vi "parse alarms string.vi"(0 "Alarms String":string) -> (4 "Description":string[](array[string]), 5 "Date":string[](array[string]), 6 "Alarm Level":string[](array[string]), 7 "Alarmed Variables":string[](array[string]), 8 "Alarmed Variable Value":string[](array[string]))   [LabVIEW 2013]
panel:
  out "Array":string[](array[string])
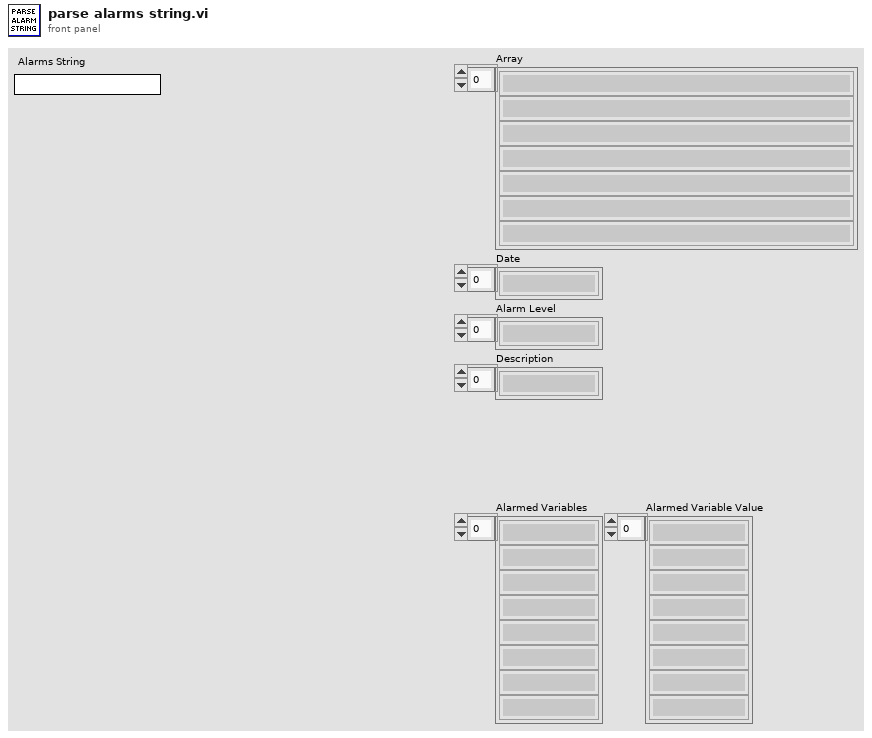
[diagram p1: front panel]
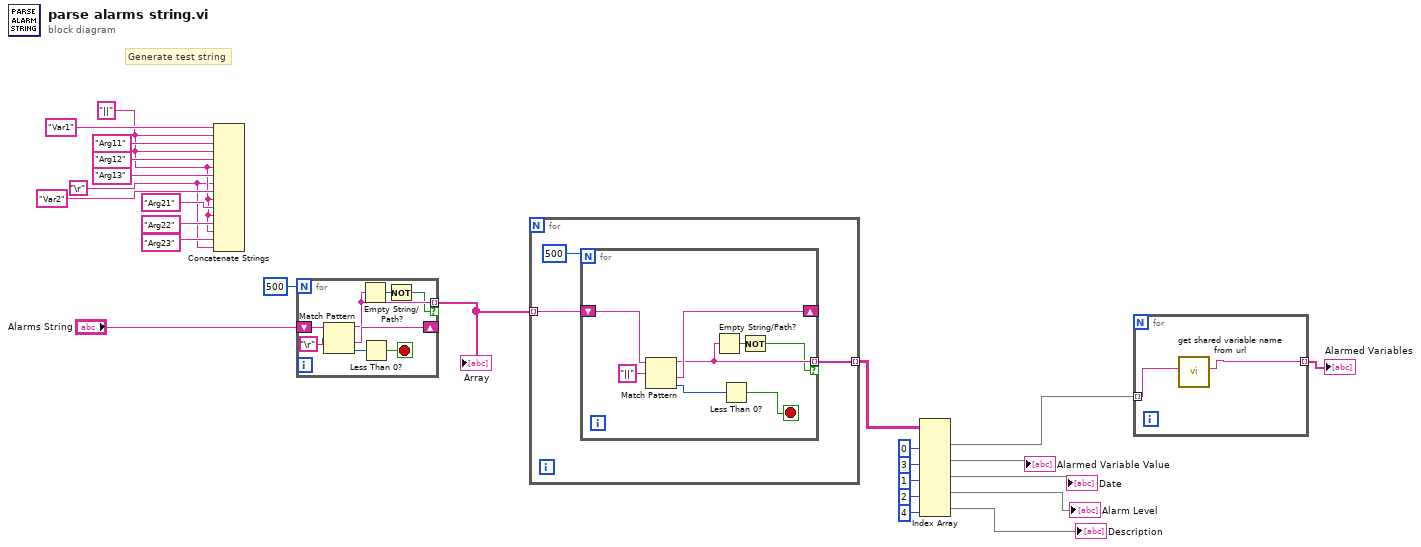
[diagram p0: block diagram]
diagram:
  w17 = "||"
  w15 = "\r"
  # "Generate test string"
  n1 = Concatenate Strings("Var1" ("string"), w17, "Arg11" ("string"), w17, "Arg12" ("string"), w17, "Arg13" ("string"), w15, "Var2" ("string"), w17, "Arg21" ("string"), w17, "Arg22" ("string"), w17, "Arg23" ("string"), w15) -> ()  [unwired: 1 out]
  n2 = for {
    N: 500 -> [_]
    shift-right: [w30] -> _
    shift-left: "Alarms String" -> [w33]
    tunnel: [w27] -> w25 mode=indexing if=w26
    stop <- w31 stop-if-true
    n3 = Match Pattern(string=w33, regular expression="\r") -> (before substring=w27:string, after substring=w30:string, offset past match=w32:i32)  [unwired: 1 in, 1 out]
    n4 = Empty String/Path?(string/path=w27) -> (empty?=w28:bool)
    n5 = Less Than 0?(x=w32) -> (x < 0?=w31:bool)
    n6 = Not(x=w28) -> (.not. x?=w26:bool)
  }
  "Array" <- w25
  n7 = for {
    tunnel: w25 -> [w36] mode=indexing
    tunnel: [w34] -> w13 mode=indexing
    n8 = for {
      N: 500 -> [_]
      shift-right: [w40] -> _
      shift-left: w36 -> [w44]
      tunnel: [w39] -> w34 mode=indexing if=w37
      stop <- w41 stop-if-true
      n9 = Match Pattern(string=w44, regular expression="||") -> (before substring=w39:string, after substring=w40:string, offset past match=w42:i32)  [unwired: 1 in, 1 out]
      n10 = Empty String/Path?(string/path=w39) -> (empty?=w38:bool)
      n11 = Less Than 0?(x=w42) -> (x < 0?=w41:bool)
      n12 = Not(x=w38) -> (.not. x?=w37:bool)
    }
  }
  n13 = Index Array(array=w13, index (col) #1=0 ("disabled index (col)"), index (col) #2=3 ("index (col)"), index (col) #3=1 ("index (col)"), index (col) #4=2 ("index (col)"), index (col) #5=4 ("index (col)")) -> (element #1=w8:string[], element #2=→"Alarmed Variable Value":string[], element #3=→"Date":string[], element #4=→"Alarm Level":string[], element #5=→"Description":string[])  [unwired: 5 in]
  n14 = for {
    tunnel: w8 -> [w46] mode=indexing
    tunnel: [w45] -> w7 mode=indexing
    n15 = call "get shared variable name from url.vi"("string in"=w46) -> ("Shared Variable"=w45:string)  [unwired: 9 in, 1 out]
  }
  "Alarmed Variables" <- w7
